vi "RT_Velocity mode_Oct 25_R3.vi"() -> ()   [LabVIEW 2018]
uses:
  <vilib>/Platform/TimedLoop/XDataNode/XDataNode.xnode
  <vilib>/Platform/TimedLoop/XDataNode/nitl_modes.ctl
  <vilib>/Platform/TimedLoop/XDataNode/XDNodeRunTimeDep.lvlib
  <vilib>/Platform/TimedLoop/XDataNode/wakeup.ctl
  <vilib>/Platform/TimedLoop/XDataNode/timing_clust.ctl
  <vilib>/rvi/interface/nirviReadWriteControl/nirviReadWriteControl.xnode
  Type Defs/BL Measurement States.ctl
  <vilib>/rvi/interface/nirviCloseFPGA/nirviCloseFPGA.xnode
  <vilib>/FPGAPlugInAG/Dynamic/niLvFpga_Close_Dynamic.vi
  <vilib>/rvi/interface/nirviOpenFPGA/nirviOpenFPGA.xnode
  NiFpgaLv.dll
  <vilib>/Utility/error.llb/Error Cluster From Error Code.vi
  <vilib>/rvi/interface/Simulation/niFpgaSimulationCallBeginRW.vi
  <vilib>/rvi/errors/niLvFpgaAdjustHostInterfaceError.vi
  UNCC Watt balance Oct19/FPGA Bitfiles/UNCCWattbalanceO_FPGATarget_fpganestedFORW&R_aHmrZ4eE-L4.lvbitx
  FPGA files/fpga_nestedFOR_W&R_ADC_W_2DACs_Write_then_CLK.vi
  <vilib>/FPGAPlugInAG/myRIO-1900/niLvFpga_Open_myRIO-1900.vi
  <vilib>/rvi/interface/common/dynamic/niFpgaDynamicAddResources.vi
panel:
  out "Late":bool
  out "Queue On":bool
  out "BL":dbl=14.310883864096947
  out "Numeric Control":i32
  out "Velocity (m/s)":dbl=0.03333406380742028
  out "raw BL":dbl
  out "Lissajou":cluster{dbl[], dbl[]}(graph) caption="XY Graph - dark"
  in  "Measure":bool
  in  "reset BL":bool
  in  "no. data points":u16=500
  in  "Period (us)":i64=200
  in  "EMF Gain":dbl=1.0
  in  "offset (V)":dbl format="%#_13g"
  in  "frequency (Hz)":dbl=27.0 format="%#_13g"
  in  "amplitude (V)":dbl=0.4 format="%#_13g"
  in  "Stop Button":bool
  out "?":cluster{dbl, dbl}(graph)={161.59573981109904, -162.80879503181404}
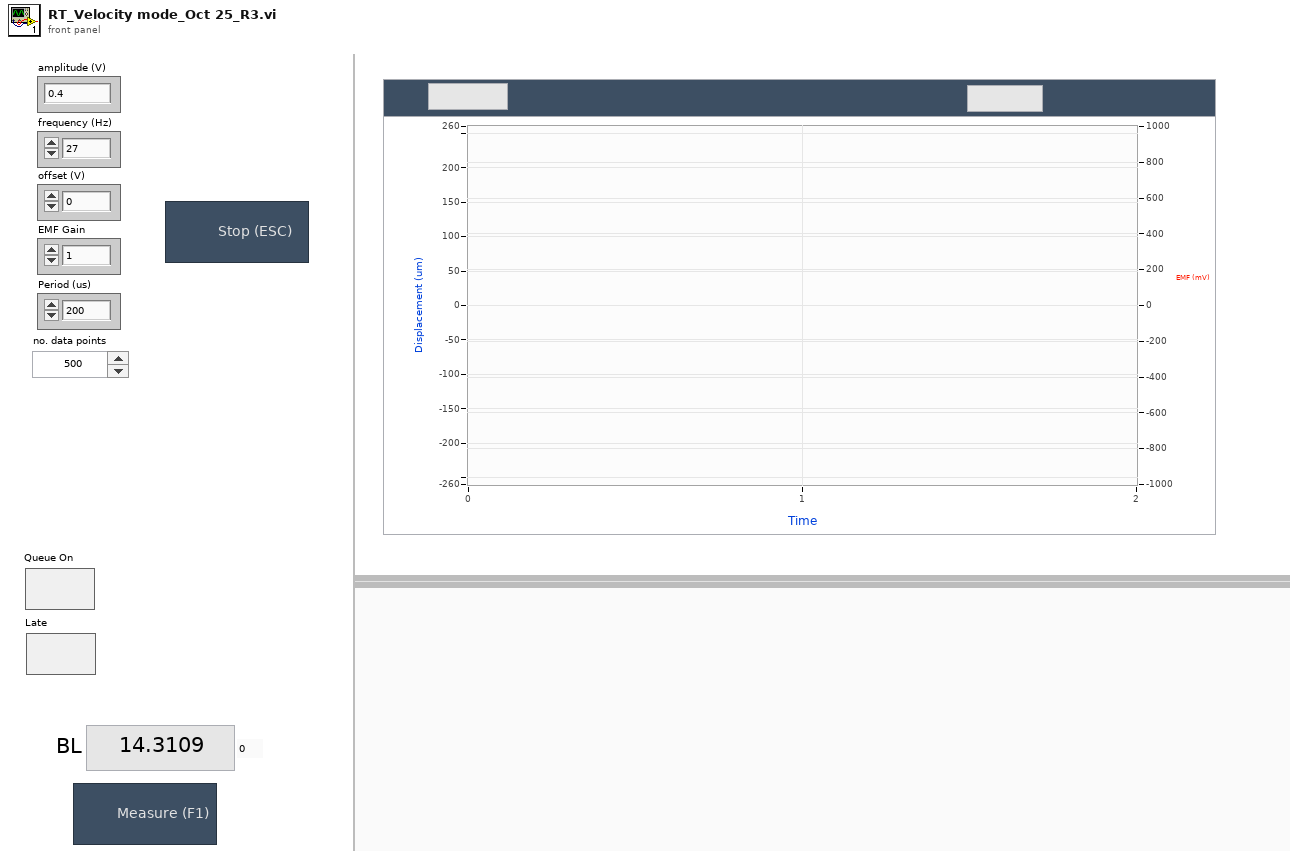
[diagram p1: front panel]
types:
  T1 = typedef "BL Measurement States.ctl" = enum16{"reset BL avg", "idle", "initialize", "collect data", "prepare data", "fit sine", "calculate BL", "exit meas"}
  T2 = typedef "XDNodeRunTimeDep.lvlib/timing_clust.ctl" = cluster{"Expected End [f-1]":u64, "Actual End [f-1]":u64, "Finished Late? [f-1]":bool, "Expected End [i-1]":u64, "Actual End [i-1]":u64, "Finished Late? [i-1]":bool, "Expected Start [i]":u64, "Actual Start [i]":u64, "Expected Start [f]":u64, "Actual Start [f]":u64, "Source Name":string, "Structure Name":string, "Period":i64, "Deadline":i64, "Offset":i64, "Start":i64, "Priority":i32, "Timeout":i32, "Mode":T3, "Wakeup Reason":T4, "Error":errorcluster, "Source Type":string, "Secondary Source Type":string, "Global End Time":u64, "Global Start Time":u64, "Frame Duration":u64, "Iteration Duration":u64, "Assigned CPU":i32, "I/O Scan Engine Mode":u32}
  T3 = typedef "XDNodeRunTimeDep.lvlib/nitl_modes.ctl" = enum32{"No Change", "Process missed periods, maintain original phase", "Discard missed periods, maintain original phase", "Process missed periods, ignore original phase", "Discard missed periods, ignore original phase"}
  T4 = typedef "XDNodeRunTimeDep.lvlib/wakeup.ctl" = enum32{"Normal", "Aborted", "Asynchronous wakeup", "Timing source error", "Timed loop error", "Timeout"}
  T5 = typedef "Fourier Outputs.ctl" = cluster{"Time period":dbl, "computed \namplitude":dbl, "number of cycles":dbl}
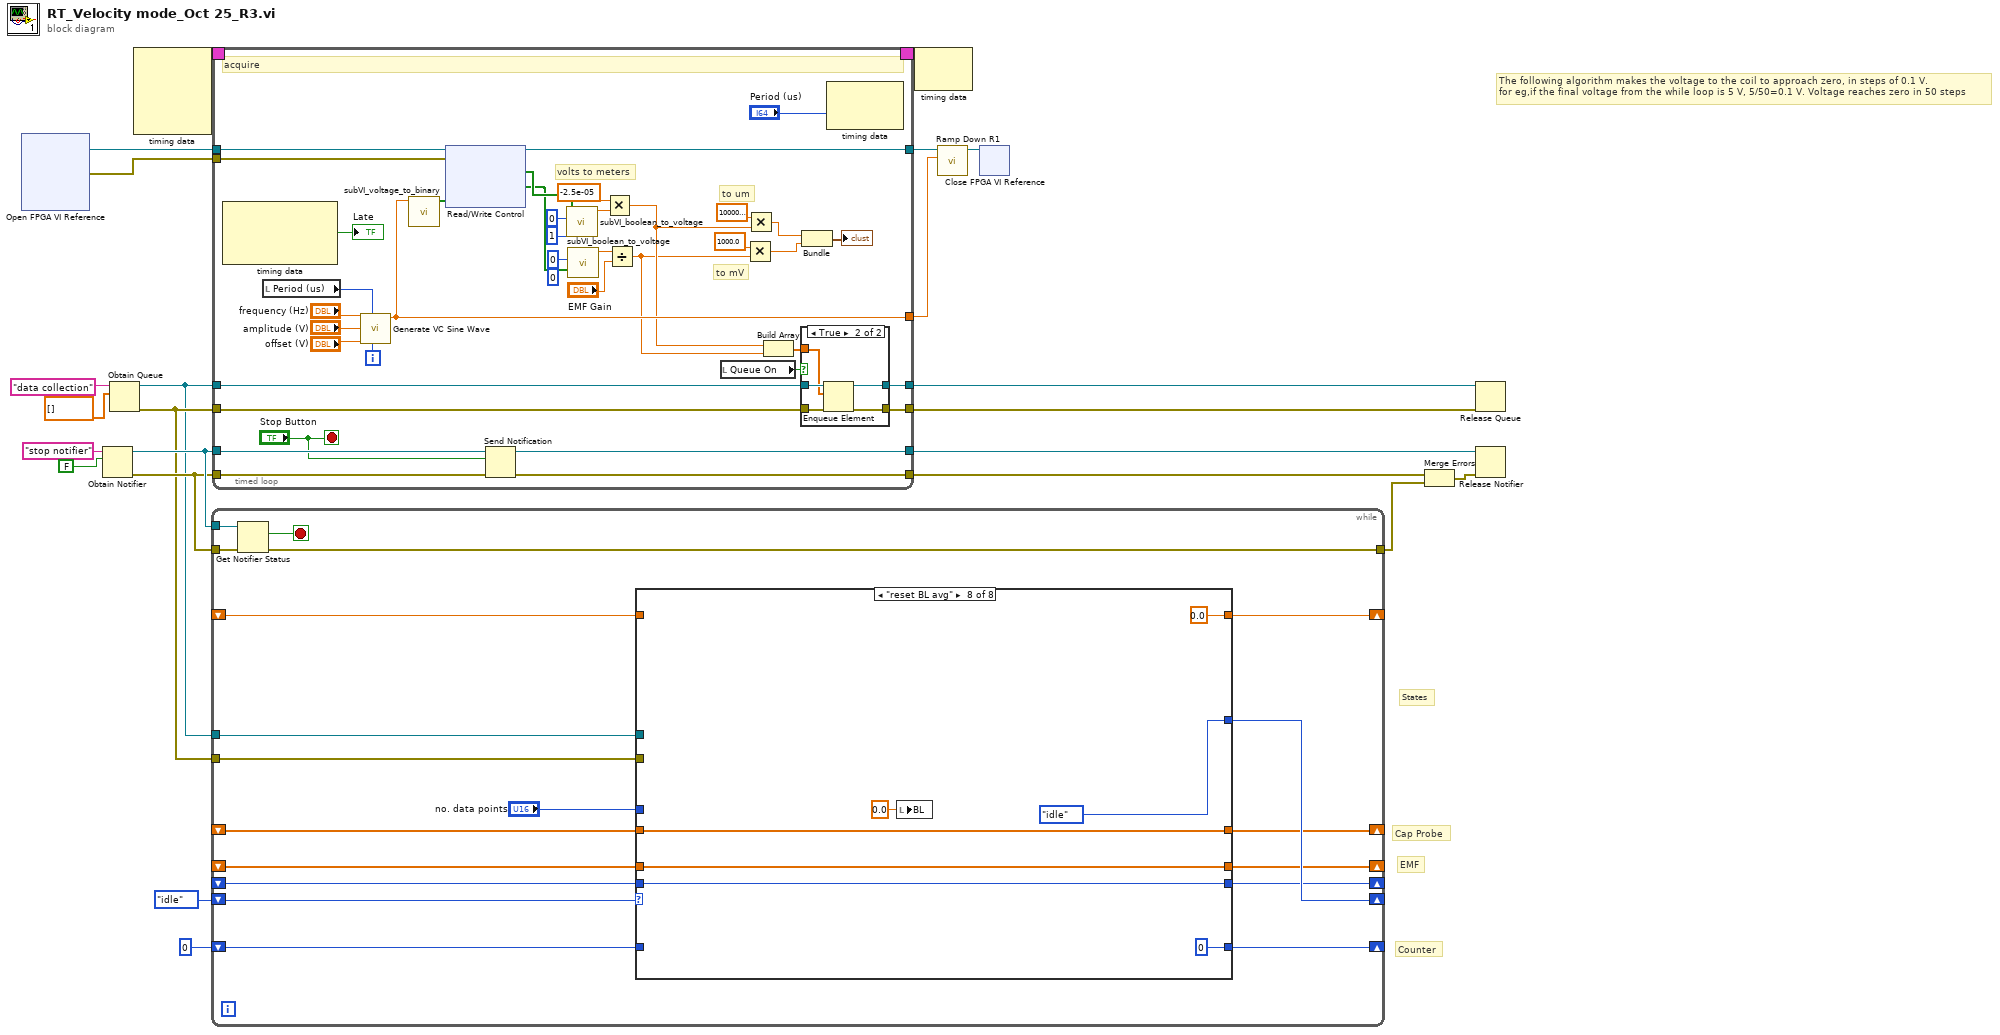
[diagram p0: block diagram]
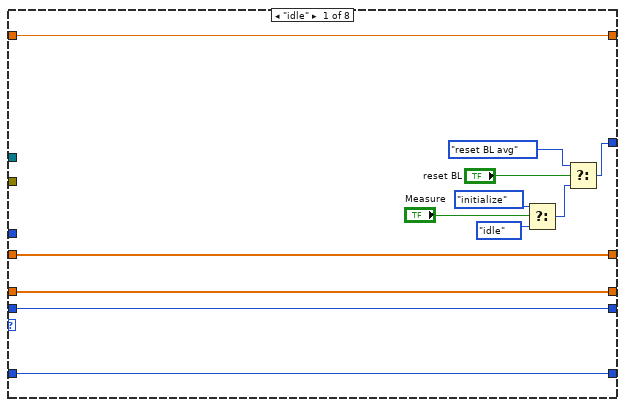
[diagram p2: hidden frame]
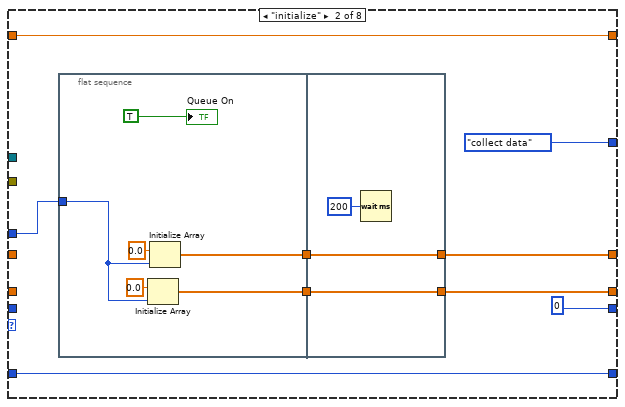
[diagram p3: hidden frame]
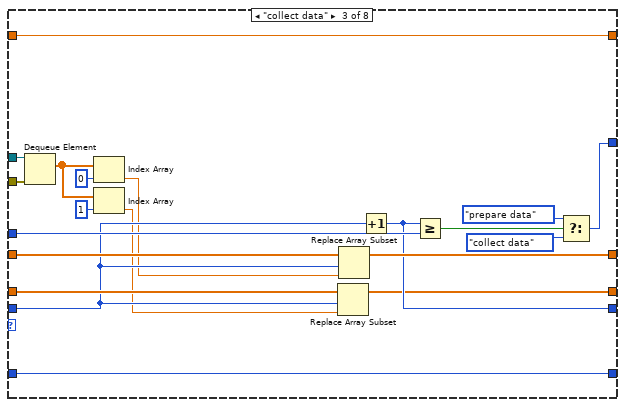
[diagram p4: hidden frame]
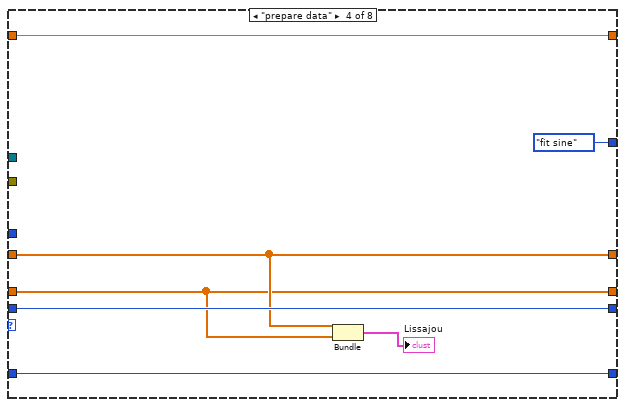
[diagram p5: hidden frame]
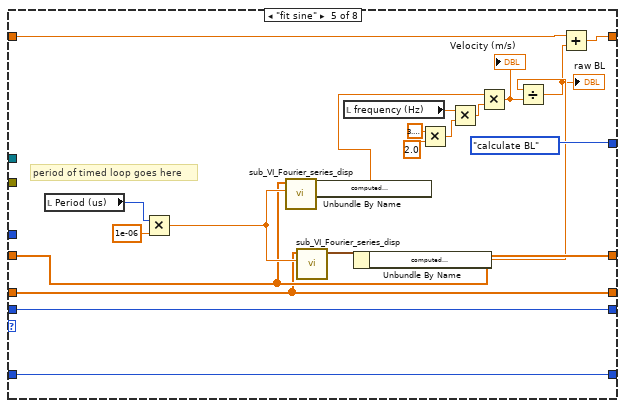
[diagram p6: hidden frame]
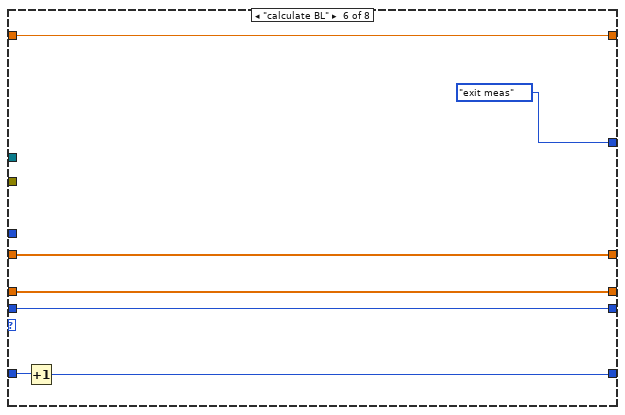
[diagram p7: hidden frame]
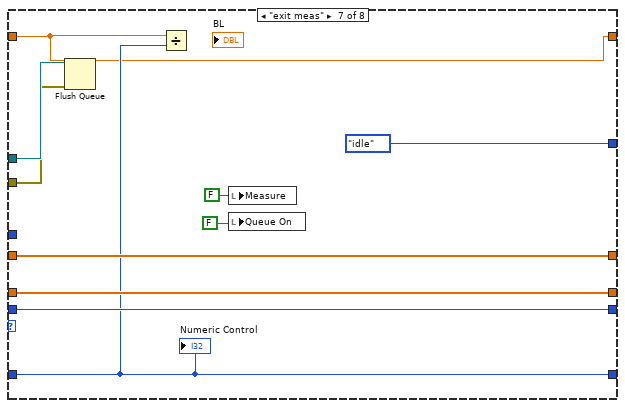
[diagram p8: hidden frame]
diagram:
  # "The following algorithm makes the voltage to the coil to approach zero, in steps of 0.1 V.\nfor eg,if the final voltage from the while loop is 5 V, 5/50=0.1 V. Voltage reaches zero in 50 steps"
  # "States"
  # "Counter"
  # "EMF"
  # "Cap Probe"
  n1 = xnode "Open FPGA VI Reference"() -> ("FPGA VI Reference Out"=w3:refnum<k20>, "error out"=w2:errorcluster)  [unwired: 2 in]
  n2 = Obtain Notifier(name (unnamed)="stop notifier", notification data type=FALSE) -> (notifier out=w15:refnum<notifier>, error out=w14:errorcluster)  [unwired: 2 in, 1 out]
  n3 = Obtain Queue(name (unnamed)="data collection", element data type=dbl[] [] ("appended array")) -> (queue out=w4:refnum<queue>, error out=w5:errorcluster)  [unwired: 3 in, 1 out]
  n4 = node-c288() -> (w23:T2)  [unwired: 4 in]
  n5 = while {
    shift-right: [w36] -> _
    shift-left: 0 -> [w32]
    shift-right: [w37] -> _
    shift-left: _ -> [w33]
    shift-right: [w38] -> _
    shift-left: _ -> [w34]
    shift-right: [w39] -> _
    shift-left: _ -> [w35]
    shift-right: [w41] -> _
    shift-left: _ -> [w42]
    shift-right: [w40] -> _
    shift-left: BL_Measurement_States."idle" ("BL meas states") -> [w26]
    tunnel: w15 -> [w30]
    tunnel: w14 -> [w29]
    tunnel: [w27] -> w12
    tunnel: w5 -> [w24]
    tunnel: w4 -> [w25]
    stop <- w28 stop-if-true
    n6 = Get Notifier Status(notifier=w30, error in (no error)=w29) -> (current notification=w28:bool, error out=w27:errorcluster)  [unwired: 3 out]
    n7 = case shown="\"reset BL avg\"" w26 {
      tunnel: [w45 BL_Measurement_States."collect data" ("BL meas states") w86 BL_Measurement_States."fit sine" ("BL meas states") BL_Measurement_States."calculate BL" ("BL meas states") BL_Measurement_States."exit meas" ("BL meas states") BL_Measurement_States."idle" ("BL meas states") BL_Measurement_States."idle" ("BL meas states")] -> w40
      tunnel: [w50 w61 w87 w95 w113 w127 w136 w143] -> w39
      tunnel: [w49 w60 w83 w93 w112 w125 w133 w142] -> w38
      tunnel: w35 -> [w50 _ w89 w95 w113 w127 w136 w143]
      tunnel: w33 -> [w51 _ w82 w99 w120 w126 w135 w141]
      tunnel: [w51 0 w85 w99 w120 w126 w135 w141] -> w37
      tunnel: "no. data points" -> [_ w59 w88 _ _ _ _ _]
      tunnel: w34 -> [w49 _ w84 w93 w112 w125 w133 w142]
      tunnel: [w43 w58 w81 w97 w111 w123 w131 0.0] -> w41
      tunnel: w42 -> [w43 w58 w81 w97 w110 w123 w131 _]
      tunnel: w32 -> [w44 w57 w80 w96 w109 w124 w132 _]
      tunnel: [w44 w57 w80 w96 w109 w122 w132 0] -> w36
      tunnel: w25 -> [_ _ w79 _ _ _ w130 _]
      tunnel: w24 -> [_ _ w78 _ _ _ w129 _]
      frame "idle" {
        n8 = Select(t=BL_Measurement_States."initialize" ("BL meas states"), s="Measure", f=BL_Measurement_States."idle" ("BL meas states 2")) -> (s? t:f=w46:T1)
        n9 = Select(t=BL_Measurement_States."reset BL avg" ("BL meas states"), s="reset BL", f=w46) -> (s? t:f=w45:T1)
      }
      frame "initialize" {
        n10 = flat-sequence {
          tunnel: w59 -> [w67]
          tunnel: [w69] -> w56
          tunnel: [w68] -> w55
          tunnel: [w71] -> w60
          tunnel: [w72] -> w61
          tunnel: w56 -> [w72]
          tunnel: w55 -> [w71]
          frame #0 {
            n11 = Initialize Array(0.0 ("element"), w67) -> (w68:dbl[])
            n12 = Initialize Array(0.0 ("element"), w67) -> (w69:dbl[])
            "Queue On" <- TRUE
          }
          frame #1 {
            n13 = Wait (ms)(milliseconds to wait=u32 200) -> ()  [unwired: 1 out]
          }
        }
      }
      frame "collect data" {
        n14 = Dequeue Element(queue=w79, error in (no error)=w78) -> (element=w77:dbl[])  [unwired: 1 in, 3 out]
        n15 = Index Array(array=w77, index=0) -> (element=w74:dbl)
        n16 = Index Array(array=w77, index=1) -> (element=w73:dbl)
        n17 = Replace Array Subset(array=w84, new element=w73, index=w82) -> (w83:dbl[])
        n18 = Replace Array Subset(array=w89, new element=w74, index=w82) -> (w87:dbl[])
        n19 = Increment(x=w82) -> (x+1=w85:i32)
        n20 = Greater Or Equal?(x=w85, y=w88) -> (x >= y?=w90:bool)
        n21 = Select(t=BL_Measurement_States."prepare data" ("BL meas states"), s=w90, f=BL_Measurement_States."collect data" ("BL meas states 2")) -> (s? t:f=w86:T1)
      }
      frame "prepare data" {
        n22 = Bundle(w95, w93) -> (→"Lissajou":cluster{dbl[], dbl[]})  [unwired: 1 in]
      }
      frame "fit sine" {
        # "period of timed loop goes here"
        n23 = local read "Period (us)"() -> (w108:i64)
        n24 = Multiply(x=w108, y=1e-06) -> (x*y=w114:dbl)
        n25 = call "sub_VI_Fourier_series_disp.vi"("del t"=w114, "x,i"=w113) -> ("outputs"=w107:T5)  [unwired: 8 in, 1 out]
        n26 = Unbundle By Name(w107) -> ("computed \namplitude"=w105:dbl)
        n27 = call "sub_VI_Fourier_series_disp.vi"("del t"=w114, "x,i"=w112) -> ("outputs"=w106:T5)  [unwired: 8 in, 1 out]
        n28 = local read "frequency (Hz)"() -> (w104:dbl)
        n29 = Unbundle By Name(w106) -> ("computed \namplitude"=w101:dbl)
        n30 = Multiply(x=3.141592653589793, y=2.0) -> (x*y=w103:dbl)
        n31 = Multiply(x=w104, y=w103) -> (x*y=w115:dbl)
        n32 = Multiply(x=w105, y=w115) -> (x*y=w102:dbl)
        "Velocity (m/s)" <- w102
        n33 = Divide(x=w101, y=w102) -> (x/y=w100:dbl)
        "raw BL" <- w100
        n34 = Add(x=w110, y=w100) -> (x+y=w111:dbl)
      }
      frame "calculate BL" {
        n35 = Increment(x=w124) -> (x+1=w122:i32)
      }
      frame "exit meas" {
        n36 = Flush Queue(queue=w130, error in (no error)=w129) -> ()  [unwired: 3 out]
        n37 = Divide(x=w131, y=w132) -> ()  [unwired: 1 out]
        n38 = local write "Measure"(FALSE) -> ()
        n39 = local write "Queue On"(FALSE) -> ()
        "Numeric Control" <- w132
      }
      frame "reset BL avg" {
        n40 = local write "BL"(0.0 ("BL")) -> ()
      }
    }
  }
  n41 = timed-loop {
    timing: w23 -> [_]
    timing-out: [_] -> w22
    tunnel: w3 -> [w163]
    tunnel: w2 -> [w177]
    tunnel: [w164] -> w20
    tunnel: [w149] -> w1
    tunnel: w15 -> [w162]
    tunnel: w14 -> [w160]
    tunnel: [w159] -> w10
    tunnel: [w158] -> w13
    tunnel: w4 -> [w155]
    tunnel: w5 -> [w154]
    tunnel: [w152] -> w7
    tunnel: [w151] -> w6
    i -> [w183]
    stop <- "Stop Button" stop-if-true
    (unwired) i16 0 ("Gain")
    # "to mV"
    # "to um"
    # "volts to meters"
    # "acquire"
    n42 = node-c288() -> (→"Late":bool)  [unwired: 1 in, 2 out]
    n43 = local read "Period (us)"() -> (w180:i64)
    n44 = call "Generate VC Sine Wave.vi"("Counter"=w183, "Period (us)"=w180, "offset (V)"="offset (V)", "amplitude (V)"="amplitude (V)", "frequency (kHz)"="frequency (Hz)") -> ("V"=w164:dbl)  [unwired: 6 in]
    n45 = call "subVI_voltage_to_binary.vi"("voltage"=w164) -> ("binary"=w145:bool[])  [unwired: 10 in]
    n46 = xnode "Read/Write Control"("FPGA VI Reference In"=w163, "error in"=w177, "DAC 1 write"=w145) -> ("FPGA VI Reference Out"=w149:refnum<k20>, "ADC  1 R"=w147:bool[], "ADC 2 R"=w146:bool[])  [unwired: 1 out]
    n47 = Send Notification(notification="Stop Button", notifier=w162, error in (no error)=w160) -> (notifier out=w159:refnum<notifier>, error out=w158:errorcluster)
    n48 = call "subVI_boolean_to_voltage.vi"("Gain"=i16 1, "UNI"=i16 0, "ADC read"=w147) -> ("V"=w173:dbl)  [unwired: 8 in]
    n49 = call "subVI_boolean_to_voltage.vi"("UNI"=i16 0, "ADC read"=w146) -> ("V"=w172:dbl)  [unwired: 9 in]
    n50 = Multiply(x=-2.5e-05, y=w173) -> (x*y=w157:dbl)
    n51 = Divide(x=w172, y="EMF Gain") -> (x/y=w156:dbl)
    n52 = local read "Queue On"() -> (w150:bool)
    n53 = Multiply(x=1000.0, y=w156) -> (x*y=w167:dbl)
    n54 = Multiply(x=1000000.0, y=w157) -> (x*y=w165:dbl)
    n55 = Build Array(w157, w156) -> (w153:dbl[])
    n56 = case shown="True" w150 {
      tunnel: w155 -> [w185 w190]
      tunnel: w154 -> [w184 w189]
      tunnel: w153 -> [_ w188]
      tunnel: [w185 w187] -> w152
      tunnel: [w184 w186] -> w151
      frame False {
      }
      frame True {
        n57 = Enqueue Element(queue=w190, element=w188, error in (no error)=w189) -> (queue out=w187:refnum<queue>, error out=w186:errorcluster)  [unwired: 1 in, 1 out]
      }
    }
    n58 = Bundle(w165, w167) -> (→"?":cluster{dbl, dbl})  [unwired: 1 in]
    n59 = node-c288("Period (us)") -> ()  [unwired: 1 in, 1 out]
  }
  n60 = node-c288(w22) -> ()  [unwired: 1 out]
  n61 = call "Ramp Down R1.vi"("V"=w20, "Refnum in"=w1) -> ("Refnum out"=w21:refnum<k20>)  [unwired: 9 in]
  n62 = xnode "Close FPGA VI Reference"("FPGA VI Reference In"=w21) -> ()  [unwired: 1 in, 1 out]
  n63 = Merge Errors(w13, w12) -> (w11:errorcluster)
  n64 = Release Queue(queue=w7, error in (no error)=w6) -> ()  [unwired: 1 in, 3 out]
  n65 = Release Notifier(notifier=w10, error in (no error)=w11) -> ()  [unwired: 1 in, 3 out]
